vi "V2fit.vi"(3 "output control":T2, 4 "data":T1, 5 "X":dbl[](array[numeric]), 6 "a":dbl[](array[numeric])) -> (0 "error out":errorcluster, 1 "f'(X,a)":dbl[][](array[numeric]), 2 "f(X,a)":dbl[](array[numeric]))   [LabVIEW 2018]
doc: "This template is the starting point for creating a model function to be passed to the Nonlinear Curve Fit.vi."
uses:
  <vilib>/gmath/NumericalOptimization/LM_output select.ctl
  <vilib>/gmath/NumericalOptimization/objective function data.ctl
  <vilib>/gmath/NI_Gmath.lvlib
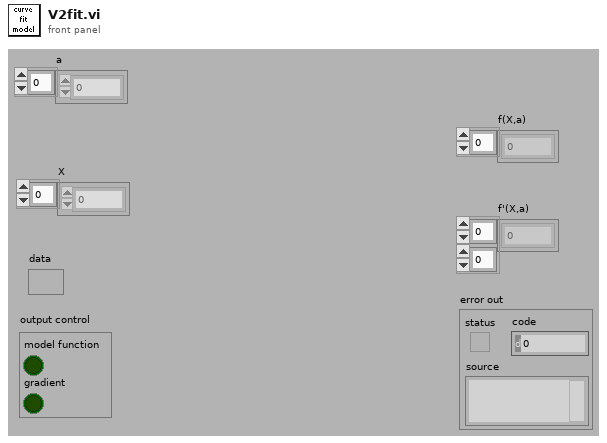
[diagram p1: front panel]
types:
  T1 = typedef "NI_Gmath.lvlib/objective function data.ctl" = variant
  T2 = typedef "NI_Gmath.lvlib/LM_output select.ctl" = cluster{"model function":bool, "gradient":bool}
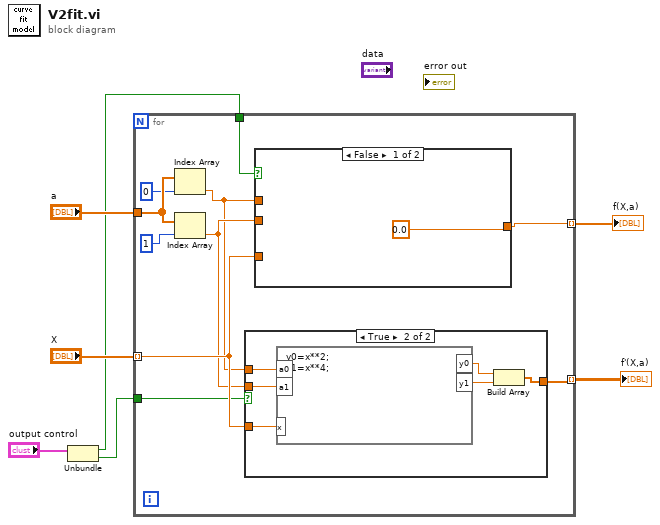
[diagram p0: block diagram]
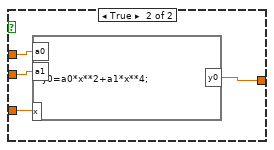
[diagram p2: hidden frame]
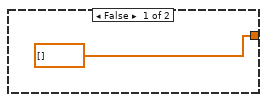
[diagram p3: hidden frame]
diagram:
  n1 = Unbundle("output control") -> ("model function"=w1:bool, "gradient"=w2:bool)
  n2 = for {
    tunnel: "a" -> [w15]
    tunnel: "X" -> [w17] mode=indexing
    tunnel: [w16] -> w5 mode=indexing
    tunnel: [w9] -> w4 mode=indexing
    tunnel: w2 -> [w10]
    tunnel: w1 -> [w8]
    n3 = Index Array(array=w15, index=0) -> (element=w11:dbl)
    n4 = Index Array(array=w15, index=1) -> (element=w12:dbl)
    n5 = case shown="True" w10 {
      tunnel: w17 -> [_ w29]
      tunnel: w12 -> [_ w28]
      tunnel: w11 -> [_ w27]
      tunnel: [dbl[] [] w24] -> w9
      frame False {
      }
      frame True {
        n6 = formula code="y0=x**2;\ny1=x**4;"("x"=w29, "a0"=w27, "a1"=w28) -> ("y0"=w25:dbl, "y1"=w26:dbl)
        n7 = Build Array(w25, w26) -> (w24:dbl[])
      }
    }
    n8 = case shown="False" w8 {
      tunnel: w17 -> [_ w22]
      tunnel: [0.0 w21] -> w16
      tunnel: w12 -> [_ w20]
      tunnel: w11 -> [_ w19]
      frame False {
      }
      frame True {
        n9 = formula code="y0=a0*x**2+a1*x**4;"("x"=w22, "a0"=w19, "a1"=w20) -> ("y0"=w21:dbl)
      }
    }
  }
  "f(X,a)" <- w5
  "f'(X,a)" <- w4
